vi "RT Driver VI.vi"(7 "Operation":T1, 11 "Device Reference in":T2 format="%.0x") -> (0 "Error Code":i32)   [LabVIEW 2013, in "FPGA Addon Engine.lvlib"]
uses:
  FPGA Addon Engine.lvlib
  <vilib>/NI Veristand/Custom Device API/Custom Device Item Ref.ctl
  <vilib>/NI Veristand/Custom Device API/Hardware Interface Driver VI Operation.ctl
  Shared/FPGA Settings.vi
  SubVIs/Initialize Scalar Datatypes and Refs.vi
  <vilib>/Utility/config.llb/Open Config Data.vi
  <vilib>/Utility/config.llb/Get Key Names.vi
  <vilib>/Utility/config.llb/Write Key.vi
  <vilib>/Utility/config.llb/Write Key (I32).vi
  <vilib>/Utility/config.llb/Close Config Data.vi
  Shared/Constants.vi
  <vilib>/NI Veristand/Custom Device API/NI VeriStand - Get Item Property.vi
  <vilib>/NI Veristand/Custom Device API/Get Item Property (Variant).vi
  <vilib>/NI Veristand/Custom Device API/NI VeriStand - Get Target Type.vi
  <vilib>/NI Veristand/Custom Device API/Get Item Property (Dependent File).vi
  SubVIs/Initialize Input DMA Refs.vi
  SubVIs/Initialize Output DMA Refs.vi
  <vilib>/NI Veristand/Custom Device API/Get Item Property (Path).vi
  <vilib>/NI Veristand/Custom Device API/Get Item Property (String).vi
  SubVIs/Initialize Scalar Datatype Classes.vi
  SubVIs/Output DMA Engine.vi
  <vilib>/rvi/interface/common/niFpgaWaitOnOcc.vi
  <vilib>/Utility/error.llb/Error Cluster From Error Code.vi
  <vilib>/RVI Host/nirviSupport.llb/nirviErrorClusterFromErrorCode.vi
  <vilib>/rvi/errors/niLvFpgaAdjustHostInterfaceError.vi
  <vilib>/NI Veristand/Custom Device API/Global Data Refs.vi
  <vilib>/FPGAPlugInAG/Dynamic/niLvFpga_Close_Dynamic.vi
  <vilib>/NI Veristand/Custom Device Waveform API/Multiple Waveforms Write (DBL)/Multiple Waveforms Write (DBL).lvclass
  <vilib>/NI Veristand/Custom Device Waveform API/Single Waveform Read (DBL)/Single Waveform Read (DBL).lvclass
  <vilib>/rvi/interface/nirviMethod/nirviMethod.xnode
  <vilib>/rvi/interface/nirviCloseFPGA/nirviCloseFPGA.xnode
  <vilib>/NI VeriStand/Custom Device API/Custom Device API.lvlib
  <vilib>/NI Veristand/Custom Device Tools/Custom Device Utility Library/Custom Device Utility Library.lvlib
  SubVIs/Inline Async API/Inline Async API.lvlib
  SubVIs/Error Handling API/Error Handling API.lvlib
  <vilib>/rvi/interface/nirviMethod/StockFPGA_InlinedMethodWaitForSingleIRQ.vi
  <vilib>/FPGAPlugInAG/Dynamic/niLvFpga_WaitOnIrq_Dynamic.vi
  <vilib>/FPGAPlugInAG/Dynamic/niLvFpga_AcknowledgeIrq_Dynamic.vi
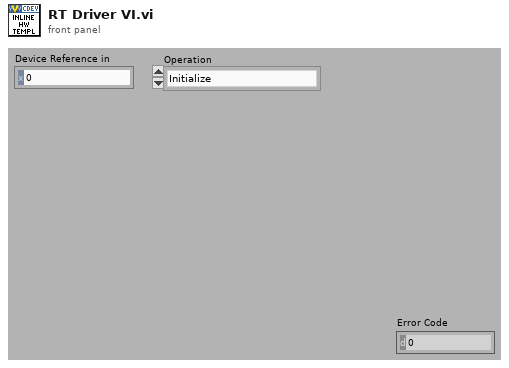
[diagram p1: front panel]
types:
  T1 = typedef "Custom Device API.lvlib/Hardware Interface Driver VI Operation.ctl" = enum16{"Initialize", "Start", "Read Data from HW", "Write Data to HW", "Close"}
  T2 = typedef "Custom Device API.lvlib/Custom Device Item Ref.ctl" = u64
  T3 = typedef "FPGA Addon Engine.lvlib/State Variables.ctl" = cluster{"FPGA Ref":refnum<k20>, "IncomingRegisters.Refs":T4[], "IncomingDMA.Refs":T7[], "OutgoingRegisters.Refs":T4[], "OutgoingDMA.Refs":T12[], "Compiled":T14}
  T4 = typedef "FPGA Addon Engine.lvlib/Register Settings.ctl" = cluster{"Data Type":T5, "U64":refnum<k20>, "U32":refnum<k20>, "U16":refnum<k20>, "U8":refnum<k20>, "I64":refnum<k20>, "I32":refnum<k20>, "I16":refnum<k20>, "I8":refnum<k20>, "SGL":refnum<k20>, "Bool":refnum<k20>, "Scalar Type":T6, "Index":i32, "Length":i32}
  T5 = typedef "Type Descriptor Enumeration__ogtk.ctl" = enum8{"<Null>", "I8", "I16", "I32", "I64", "U8", "U16", "U32", "U64", "SGL", "DBL", "EXT", "CSG", "CDB", "CXT", "0x0F", "0x10", "0x11", "0x12", "0x13", "0x14", "Enum U8", "Enum U16", "Enum U32", "Enum U64", "SGL PQ", "DBL PQ", "EXT PQ", "CSG PQ", "CDB PQ", "CXT PQ", "0x1F", "0x20", "Boolean", "0x22", "0x23", "0x24", "0x25", "0x26", "0x27", "0x28", "0x29", "0x2A", "0x2B", "0x2C", "0x2D", "0x2E", "0x2F", "String", "0x31", "Path", "Pict", "0x34", "0x35", "0x36", "DAQ", "0x38", "0x39", "0x3A", "0x3B", "0x3C", "0x3D", "0x3E", "0x3F", "Array", "0x41", "0x42", "0x43", "0x44", "0x45", "0x46", "0x47", "0x48", "0x49", "0x4A", "0x4B", "0x4C", "0x4D", "0x4E", "0x4F", "Cluster", "0x51", "0x52", "Variant", "Waveform", "0x55", "0x56", "0x57", "0x58", "0x59", "0x5A", "0x5B", "0x5C", "0x5D", "0x5E", "0x5F", "0x60", "0x61", "0x62", "0x63", "0x64", "0x65", "0x66", "0x67", "0x68", "0x69", "0x6A", "0x6B", "0x6C", "0x6D", "0x6E", "0x6F", "Refnum"}
  T6 = typedef "FPGA Addon Shared.lvlib/Scalar Type.ctl" = enum16{"Standard", "Bitpacked"}
  T7 = typedef "FPGA Addon Engine.lvlib/DMA Input References.ctl" = cluster{"Waveform Ref":refnum<class "Multiple Waveforms Write (DBL).lvclass">, "DMA Ref":T8, "Write to VS Engine.Refs":cluster{"Refs":T9[], "Values":dbl[]}, "Write to VS Engine.FIFO":refnum<k33>, "Name":string, "DMA Settings":T10}
  T8 = typedef "FPGA Addon Engine.lvlib/DMA Input Ref.ctl" = refnum<k20>
  T9 = typedef "Custom Device API.lvlib/Data Reference.ctl" = i32
  T10 = typedef "FPGA Addon Shared.lvlib/DMA Settings.ctl" = cluster{"Number of Channels":u8, "Delacing Scheme":T11, "Update Rate":u32, "dt":dbl}
  T11 = typedef "FPGA Addon Shared.lvlib/Delacing Scheme.ctl" = enum8{"Interlaced"}
  T12 = typedef "FPGA Addon Engine.lvlib/DMA Output References.ctl" = cluster{"Write to VS Engine.Refs":cluster{"Refs":T9[], "Values":dbl[]}, "Waveforms":refnum<class "Single Waveform Read (DBL).lvclass">[], "DMA Ref":T13, "Write to VS Engine.FIFO":refnum<k33>, "Name":string}
  T13 = typedef "FPGA Addon Engine.lvlib/DMA Output Ref.ctl" = refnum<k20>
  T14 = typedef "FPGA Addon Shared.lvlib/Compiled.Settings" = cluster{"Name":string, "IncomingRegisters.Settings":T15[], "IncomingRegisters.Refs":cluster{"Refs":T17[], "Values":dbl[]}, "OutgoingRegisters.Settings":T15[], "OutgoingRegisters.Refs":cluster{"Refs":T17[], "Values":dbl[]}, "Incoming.Size":i32, "Outgoing.Size":i32, "IncomingDMA.Settings":T18[], "OutgoingDMA.Settings":T18[], "FPGA.Settings":T20}
  T15 = typedef "FPGA Addon Shared.lvlib/Compiled.RegisterSettings.ctl" = cluster{"Scalar Type":T6, "Index":i32, "Length":i32, "Register":T16}
  T16 = typedef "FPGA Addon Shared.lvlib/Register Information.ctl" = cluster{"Name":string, "Data Type":T5, "Default Value":dbl}
  T17 = typedef "Custom Device API.lvlib/Block Data Reference.ctl" = cluster{"Data Reference":T9, "Offset":i32, "Length":i32}
  T18 = typedef "FPGA Addon Shared.lvlib/Compiled.DMASettings.ctl" = cluster{"Name":string, "DMA.Settings":T10, "DMA.VSRefs":T19[], "WritetoVSEngine.Refs":cluster{"Refs":T9[], "Values":dbl[]}}
  T19 = typedef "Custom Device API.lvlib/Waveform Data Reference.ctl" = i32
  T20 = typedef "FPGA Addon Shared.lvlib/FPGA Settings.ctl" = cluster{"Bitfile path":path, "RIO Device Address":string}
  T21 = typedef "FPGA Addon Engine.lvlib/Error Handling API.lvlib/Error Handling Cluster.ctl" = cluster{"Error Process Q":refnum<queue>, "Process Qs":refnum<queue>[]}
  T22 = cluster{"Vars":T3, "Async?":bool, "Async VI Refs out":refnum<vi>[], "Error Handling Refs":T21, "error out":errorcluster}
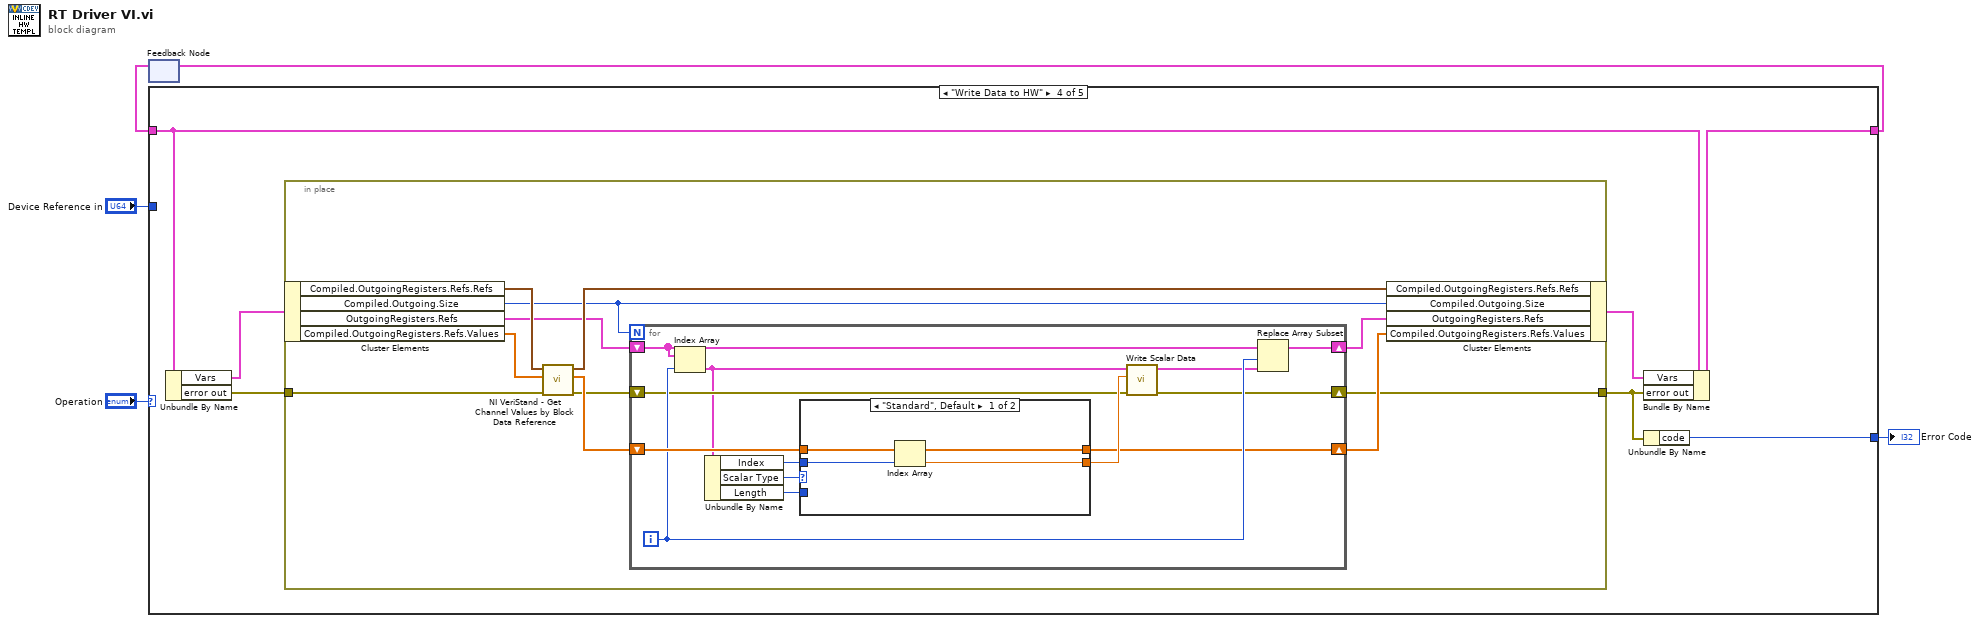
[diagram p0: block diagram]
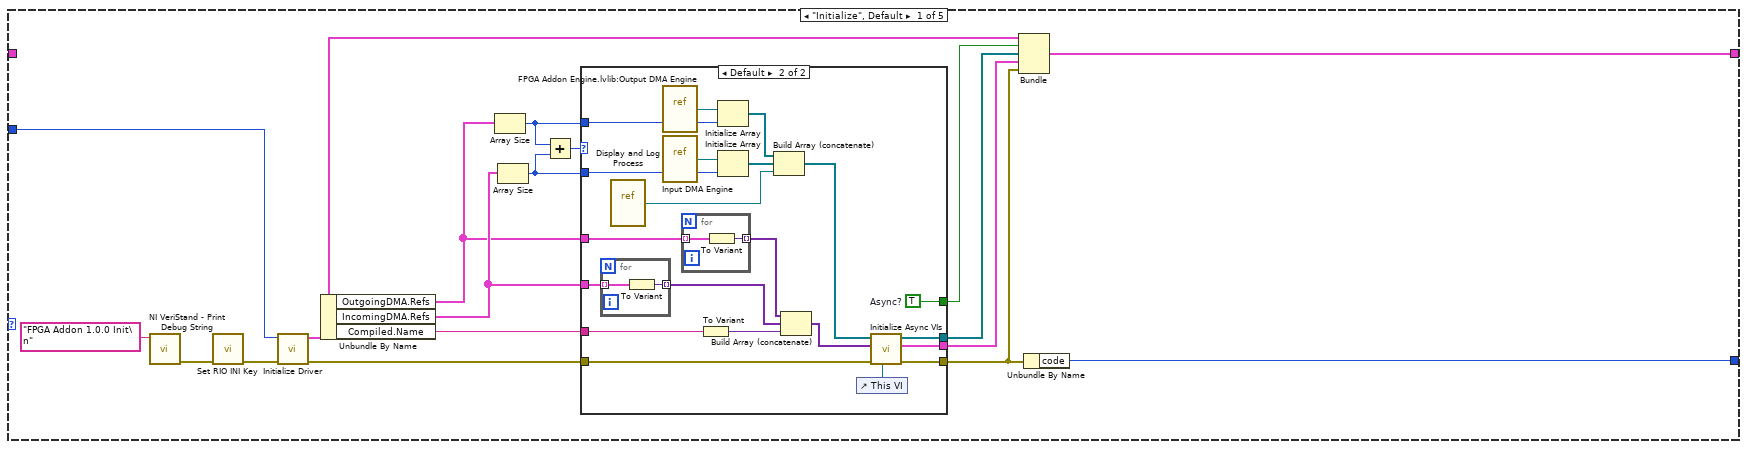
[diagram p2: hidden frame]
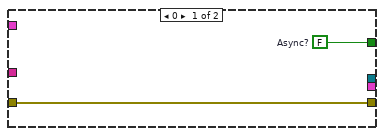
[diagram p3: hidden frame]
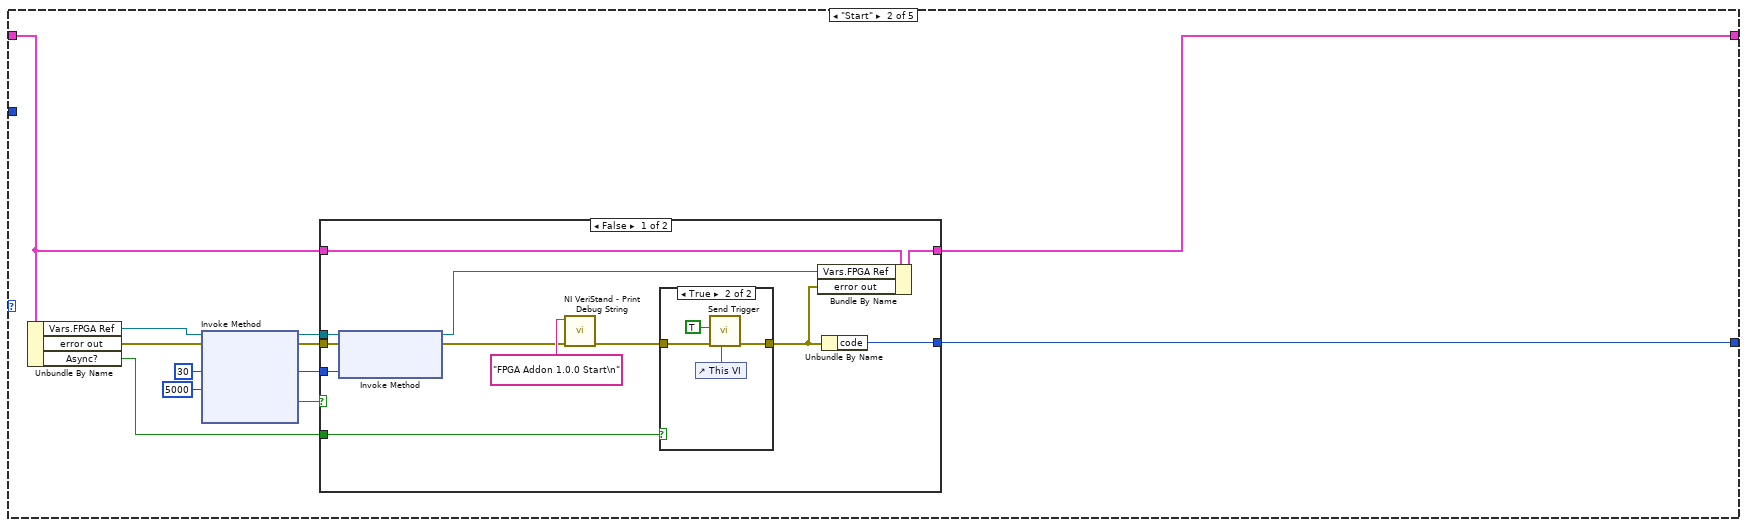
[diagram p4: hidden frame]
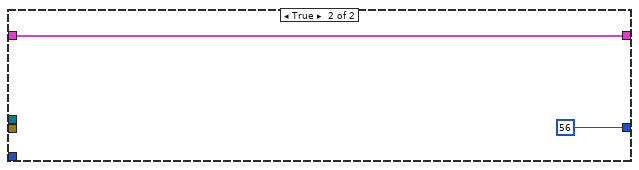
[diagram p6: hidden frame]
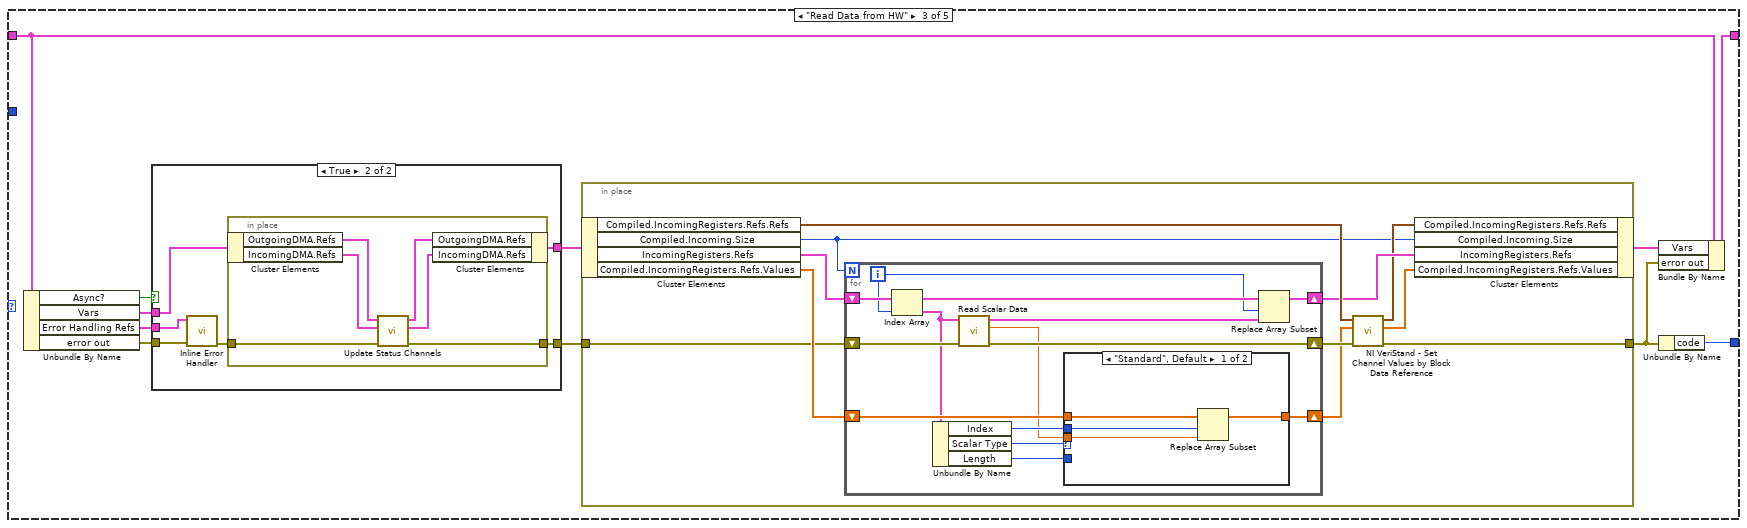
[diagram p7: hidden frame]
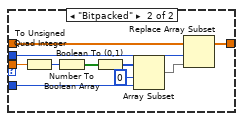
[diagram p9: hidden frame]
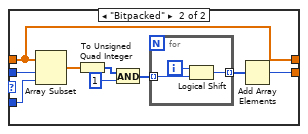
[diagram p10: hidden frame]
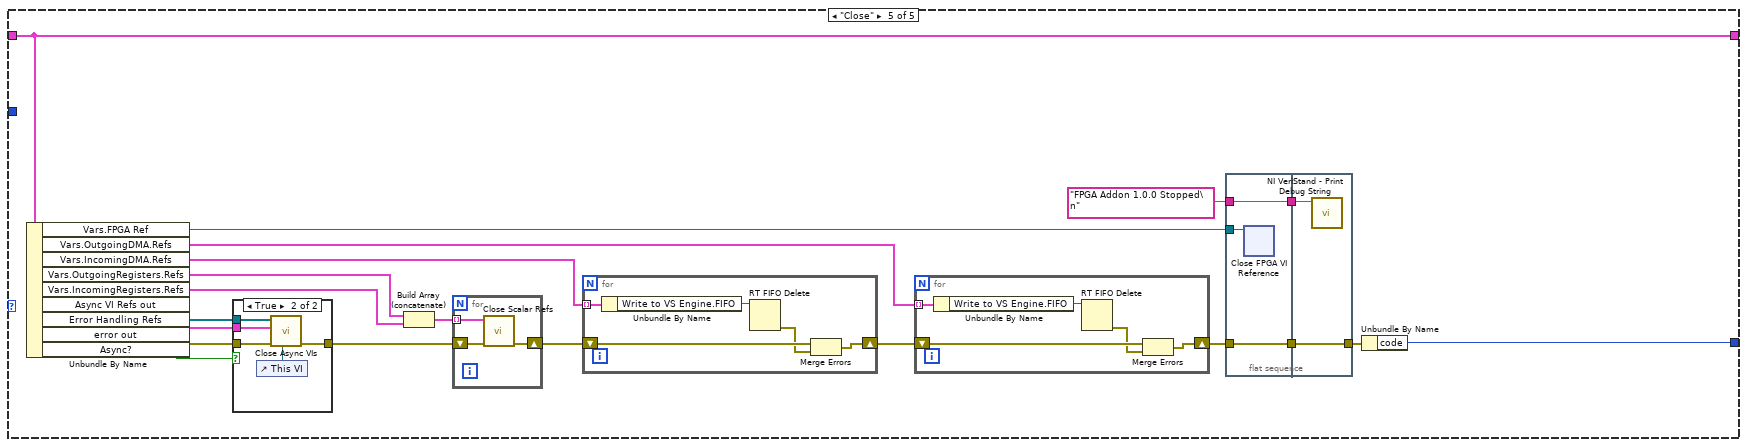
[diagram p11: hidden frame]
diagram:
  n1 = feedback #1() -> (w3:T22)  [unwired: 1 out]
  n2 = case shown="\"Write Data to HW\"" "Operation" {
    tunnel: [w23 w59 w89 w144 w207] -> w4
    tunnel: w3 -> [_ w60 w90 w145 w207]
    tunnel: "Device Reference in" -> [w21 _ _ _ _]
    tunnel: [w22 w61 w87 w146 w209] -> w1
    frame "Initialize", Default {
      n3 = call <vilib>:"NI VeriStand - Print Debug String.vi"("Message"="FPGA Addon 1.0.0 Init\n") -> ("error out"=w19:errorcluster)  [unwired: 10 in]
      n4 = call "Set RIO INI Key.vi"("error in (no error)"=w19) -> ("error out"=w18:errorcluster)  [unwired: 10 in]
      n5 = call "Initialize Driver.vi"("error in (no error)"=w18, "Section Ref in"=w21) -> ("error out"=w17:errorcluster, "Vars"=w6:T3)  [unwired: 8 in]
      n6 = Unbundle By Name(w6) -> ("OutgoingDMA.Refs"=w11:T12[], "IncomingDMA.Refs"=w13:T7[], "Compiled.Name"=w12:string)
      n7 = Array Size(array=w11) -> (size(s)=w10:i32)
      n8 = Array Size(array=w13) -> (size(s)=w9:i32)
      n9 = Add(x=w10, y=w9) -> (x+y=w8:i32)
      n10 = case shown="Default" w8 {
        tunnel: w17 -> [w25 w46]
        tunnel: [w25 w45] -> w16
        tunnel: [_ w40] -> w15
        tunnel: [_ w39] -> w14
        tunnel: w13 -> [_ w37]
        tunnel: w12 -> [_ w33]
        tunnel: w11 -> [_ w30]
        tunnel: w10 -> [_ w28]
        tunnel: w9 -> [_ w27]
        tunnel: [w24 w26] -> w7
        frame 0 {
          w24 = FALSE  # Async?
        }
        frame Default {
          w26 = TRUE  # Async?
          n11 = for {
            tunnel: w37 -> [w50] mode=indexing
            tunnel: [w49] -> w36 mode=indexing
            n12 = To Variant(anything=w50) -> (Variant=w49:variant)
          }
          n13 = vi-ref "Display and Log Process.vi"() -> (w41:refnum<vi>)
          n14 = vi-ref "FPGA Addon Engine.lvlib:Output DMA Engine.vi"() -> (w32:refnum<vi>)
          n15 = vi-ref "Input DMA Engine.vi"() -> (w44:refnum<vi>)
          n16 = for {
            tunnel: w30 -> [w48] mode=indexing
            tunnel: [w47] -> w29 mode=indexing
            n17 = To Variant(anything=w48) -> (Variant=w47:variant)
          }
          n18 = To Variant(anything=w33) -> (Variant=w35:variant)
          n19 = Initialize Array(w32, w28) -> (w31:refnum<vi>[])
          n20 = Initialize Array(w44, w27) -> (w43:refnum<vi>[])
          n21 = Build Array (concatenate)(w31, w43, w41) -> (w42:refnum<vi>[])
          n22 = Build Array (concatenate)(w29, w36, w35) -> (w34:variant[])
          n23 = control-ref of="This VI"() -> (w38:refnum<vi>)
          n24 = call "Initialize Async VIs.vi"("VI in"=w38, "error in (no error)"=w46, "Async VI Parameters"=w34, "Async VI Refs"=w42) -> ("error out"=w45:errorcluster, "Error Handling Refs"=w40:T21, "Async VI Refs out"=w39:refnum<vi>[])  [unwired: 5 in]
        }
      }
      n25 = Bundle("Vars"=w6, "Async?"=w7, "Async VI Refs out"=w14, "Error Handling Refs"=w15, "error out"=w16) -> (w23:T22)  [unwired: 1 out]
      n26 = Unbundle By Name(w16) -> ("code"=w22:i32)
    }
    frame "Start" {
      w54 = 30 ("IRQ Number(s)")
      n27 = Unbundle By Name(w60) -> ("Vars.FPGA Ref"=w58:refnum<k20>, "error out"=w57:errorcluster, "Async?"=w52:bool)
      n28 = xnode "Invoke Method"("FPGA VI Reference In"=w58, "error in"=w57, "IRQ Number(s)"=w54, "Timeout (ms)"=5000) -> ("FPGA VI Reference Out"=w56:refnum<k20>, "error out"=w55:errorcluster, "Timed Out"=w51:bool)  [unwired: 1 out]
      n29 = case shown="False" w51 {
        tunnel: [w73 56 ("code")] -> w61
        tunnel: w60 -> [w72 w80]
        tunnel: [w71 w80] -> w59
        tunnel: w56 -> [w69 _]
        tunnel: w55 -> [w68 _]
        tunnel: w54 -> [w67 _]
        tunnel: w52 -> [w62 _]
        frame False {
          n30 = xnode "Invoke Method"("FPGA VI Reference In"=w69, "error in"=w68, "IRQ Number(s)"=w67) -> ("FPGA VI Reference Out"=w66:refnum<k20>, "error out"=w65:errorcluster)
          n31 = call <vilib>:"NI VeriStand - Print Debug String.vi"("error in (no error)"=w65, "Message"="FPGA Addon 1.0.0 Start\n") -> ("error out"=w64:errorcluster)  [unwired: 9 in]
          n32 = case shown="True" w62 {
            tunnel: w64 -> [w74 w76]
            tunnel: [w74 w75] -> w63
            frame False {
            }
            frame True {
              n33 = control-ref of="This VI"() -> (w78:refnum<vi>)
              n34 = call "Send Trigger.vi"("Parent VI"=w78, "error in (no error)"=w76, "notification"=TRUE) -> ("error out"=w75:errorcluster)  [unwired: 8 in]
            }
          }
          n35 = Bundle By Name(cluster=w72, "Vars.FPGA Ref"=w66, "error out"=w63) -> (w71:T22)
          n36 = Unbundle By Name(w63) -> ("code"=w73:i32)
        }
        frame True {
        }
      }
    }
    frame "Read Data from HW" {
      n37 = Unbundle By Name(w90) -> ("Async?"=w81:bool, "Vars"=w84:T3, "Error Handling Refs"=w85:T21, "error out"=w86:errorcluster)
      n38 = case shown="True" w81 {
        tunnel: w86 -> [w93 w99]
        tunnel: w85 -> [_ w98]
        tunnel: w84 -> [w92 w97]
        tunnel: [w92 w96] -> w83
        tunnel: [w93 w94] -> w82
        frame False {
        }
        frame True {
          n39 = call "Inline Error Handler.vi"("error in"=w99, "Error Handling Cluster"=w98) -> ("error out"=w95:errorcluster)  [unwired: 9 in]
          n40 = in-place {
            in-place-border: [w101] -> w94
            in-place-border: w95 -> [w100]
            n41 = in-place-cluster #2(w97) -> ("OutgoingDMA.Refs"=w103:T12[], "IncomingDMA.Refs"=w105:T7[])
            n42 = call "Update Status Channels.vi"("error in (no error)"=w100, "DMA Input Settings"=w105, "DMA Output Settings"=w103) -> ("error out"=w101:errorcluster, "DMA Input Settings"=w104:T7[], "DMA Output Settings"=w102:T12[])  [unwired: 6 in]
            n43 = in-place-cluster #2("OutgoingDMA.Refs"=w102, "IncomingDMA.Refs"=w104) -> (w96:T3)
          }
        }
      }
      n44 = in-place {
        in-place-border: w82 -> [w107]
        in-place-border: [w109] -> w88
        n45 = in-place-cluster #3(w83) -> ("Compiled.IncomingRegisters.Refs.Refs"=w113:T17[], "Compiled.Incoming.Size"=w108:i32, "IncomingRegisters.Refs"=w116:T4[], "Compiled.IncomingRegisters.Refs.Values"=w115:dbl[])
        n46 = for {
          N: w108 -> [_]
          shift-right: [w128] -> w106
          shift-left: w115 -> [w129]
          shift-right: [w127] -> w112
          shift-left: w116 -> [w126]
          shift-right: [w124] -> w114
          shift-left: w107 -> [w125]
          i -> [w119]
          n47 = Index Array(array=w126, index=w119) -> (element=w122:T4)
          n48 = Unbundle By Name(w122) -> ("Index"=w120:i32, "Scalar Type"=w121:T6, "Length"=w118:i32)
          n49 = call "Read Scalar Data.vi"("error in (no error)"=w125, "Cluster"=w122) -> ("error out"=w124:errorcluster, "Value"=w117:dbl, "Cluster"=w123:T4)  [unwired: 7 in]
          n50 = case shown="\"Standard\", Default" w121 {
            tunnel: w129 -> [w133 w138]
            tunnel: [w132 w137] -> w128
            tunnel: w117 -> [w131 w143]
            tunnel: w120 -> [w130 w135]
            tunnel: w118 -> [_ w139]
            frame "Standard", Default {
              n51 = Replace Array Subset(array=w133, new element=w131, index=w130) -> (w132:dbl[])
            }
            frame "Bitpacked" {
              n52 = To Unsigned Quad Integer(1:w143) -> (0:w141:u64)
              n53 = Number To Boolean Array(number=w141) -> (Boolean array=w142:bool[])
              n54 = Boolean To (0,1)(Boolean=w142) -> (0, 1=w140:i16[])
              n55 = Array Subset(array=w140, index=0, length=w139) -> (w136:i16[])
              n56 = Replace Array Subset(array=w138, new element=w136, index=w135) -> (w137:dbl[])
            }
          }
          n57 = Replace Array Subset(array=w126, new element=w123, index=w119) -> (w127:T4[])
        }
        n58 = call <vilib>:"NI VeriStand - Set Channel Values by Block Data Reference.vi"("error in (no error)"=w114, "Values Array in"=w106, "Block Data Ref"=w113) -> ("error out"=w109:errorcluster, "Values Array out"=w110:dbl[], "Block Data Ref dup"=w111:T17[])  [unwired: 6 in]
        n59 = in-place-cluster #3("Compiled.IncomingRegisters.Refs.Refs"=w111, "Compiled.Incoming.Size"=w108, "IncomingRegisters.Refs"=w112, "Compiled.IncomingRegisters.Refs.Values"=w110) -> (w91:T3)
      }
      n60 = Bundle By Name(cluster=w90, "Vars"=w91, "error out"=w88) -> (w89:T22)
      n61 = Unbundle By Name(w88) -> ("code"=w87:i32)
    }
    frame "Write Data to HW" {
      n62 = Unbundle By Name(w145) -> ("Vars"=w149:T3, "error out"=w147:errorcluster)
      n63 = in-place {
        in-place-border: w147 -> [w152]
        in-place-border: [w155] -> w150
        n64 = in-place-cluster #4(w149) -> ("Compiled.OutgoingRegisters.Refs.Refs"=w161:T17[], "Compiled.Outgoing.Size"=w157:i32, "OutgoingRegisters.Refs"=w159:T4[], "Compiled.OutgoingRegisters.Refs.Values"=w154:dbl[])
        n65 = call <vilib>:"NI VeriStand - Get Channel Values by Block Data Reference.vi"("error in (no error)"=w152, "Values Array in"=w154, "Block Data Ref"=w161) -> ("error out"=w151:errorcluster, "Values Array out"=w153:dbl[], "Block Data Ref dup"=w160:T17[])  [unwired: 6 in]
        n66 = for {
          N: w157 -> [_]
          shift-right: [w162] -> w156
          shift-left: w153 -> [w172]
          shift-right: [w174] -> w158
          shift-left: w159 -> [w173]
          shift-right: [w167] -> w155
          shift-left: w151 -> [w168]
          i -> [w171]
          n67 = Index Array(array=w173, index=w171) -> (element=w166:T4)
          n68 = Unbundle By Name(w166) -> ("Index"=w164:i32, "Scalar Type"=w165:T6, "Length"=w163:i32)
          n69 = case shown="\"Standard\", Default" w165 {
            tunnel: w172 -> [w175 w178]
            tunnel: w164 -> [w177 w186]
            tunnel: [w176 w179] -> w170
            tunnel: w163 -> [_ w185]
            tunnel: [w175 w178] -> w162
            frame "Standard", Default {
              n70 = Index Array(array=w175, index=w177) -> (element=w176:dbl)
            }
            frame "Bitpacked" {
              n71 = Array Subset(array=w178, index=w186, length=w185) -> (w180:dbl[])
              n72 = To Unsigned Quad Integer(1:w180) -> (0:w181:u64[])
              n73 = And(x=w181, y=u64 1) -> (x .and. y?=w183:u64[])
              n74 = for {
                tunnel: w183 -> [w189] mode=indexing
                tunnel: [w187] -> w184 mode=indexing
                i -> [w188]
                n75 = Logical Shift(y=w188, x=w189) -> (x << y=w187:u64)
              }
              n76 = Add Array Elements(numeric array=w184) -> (sum=w179:u64)
            }
          }
          n77 = call "Write Scalar Data.vi"("error in (no error)"=w168, "Value"=w170, "Cluster"=w166) -> ("error out"=w167:errorcluster, "Cluster"=w169:T4)  [unwired: 7 in]
          n78 = Replace Array Subset(array=w173, new element=w169, index=w171) -> (w174:T4[])
        }
        n79 = in-place-cluster #4("Compiled.OutgoingRegisters.Refs.Refs"=w160, "Compiled.Outgoing.Size"=w157, "OutgoingRegisters.Refs"=w158, "Compiled.OutgoingRegisters.Refs.Values"=w156) -> (w148:T3)
      }
      n80 = Bundle By Name(cluster=w145, "Vars"=w148, "error out"=w150) -> (w144:T22)
      n81 = Unbundle By Name(w150) -> ("code"=w146:i32)
    }
    frame "Close" {
      n82 = Unbundle By Name(w207) -> ("Vars.FPGA Ref"=w196:refnum<k20>, "Vars.OutgoingDMA.Refs"=w190:T12[], "Vars.IncomingDMA.Refs"=w195:T7[], "Vars.OutgoingRegisters.Refs"=w206:T4[], "Vars.IncomingRegisters.Refs"=w205:T4[], "Async VI Refs out"=w202:refnum<vi>[], "Error Handling Refs"=w201:T21, "error out"=w204:errorcluster, "Async?"=w193:bool)
      n83 = case shown="True" w193 {
        tunnel: w204 -> [w215 w220]
        tunnel: [w215 w219] -> w203
        tunnel: w202 -> [_ w218]
        tunnel: w201 -> [_ w217]
        frame False {
        }
        frame True {
          n84 = control-ref of="This VI"() -> (w216:refnum<vi>)
          n85 = call "Close Async VIs.vi"("TopLevel VI"=w216, "error in (no error)"=w220, "Error Handling Refs"=w217, "Async VI"=w218) -> ("error out"=w219:errorcluster)  [unwired: 7 in]
        }
      }
      n86 = Build Array (concatenate)(w206, w205) -> (w208:T4[])
      n87 = for {
        tunnel: w208 -> [w231] mode=indexing
        shift-right: [w232] -> w194
        shift-left: w203 -> [w233]
        n88 = call "Close Scalar Refs.vi"("error in (no error)"=w233, "Cluster"=w231) -> ("error out"=w232:errorcluster)  [unwired: 9 in]
      }
      n89 = for {
        shift-right: [w221] -> w192
        shift-left: w194 -> [w223]
        tunnel: w195 -> [w225] mode=indexing
        n90 = Unbundle By Name(w225) -> ("Write to VS Engine.FIFO"=w224:refnum<k33>)
        n91 = RT FIFO Delete(0:w224) -> (11:w222:errorcluster)  [unwired: 2 in]
        n92 = Merge Errors(w223, w222) -> (w221:errorcluster)
      }
      n93 = for {
        shift-right: [w210] -> w191
        shift-left: w192 -> [w212]
        tunnel: w190 -> [w214] mode=indexing
        n94 = Unbundle By Name(w214) -> ("Write to VS Engine.FIFO"=w213:refnum<k33>)
        n95 = RT FIFO Delete(0:w213) -> (11:w211:errorcluster)  [unwired: 2 in]
        n96 = Merge Errors(w212, w211) -> (w210:errorcluster)
      }
      n97 = flat-sequence {
        tunnel: "FPGA Addon 1.0.0 Stopped\n" -> [w227]
        tunnel: w191 -> [w228]
        tunnel: [w228] -> w198
        tunnel: [w227] -> w197
        tunnel: w196 -> [w226]
        tunnel: [w230] -> w200
        tunnel: w198 -> [w230]
        tunnel: w197 -> [w229]
        frame #0 {
          n98 = xnode "Close FPGA VI Reference"("FPGA VI Reference In"=w226) -> ()  [unwired: 1 in, 1 out]
        }
        frame #1 {
          n99 = call <vilib>:"NI VeriStand - Print Debug String.vi"("Message"=w229) -> ()  [unwired: 10 in, 1 out]
        }
      }
      n100 = Unbundle By Name(w200) -> ("code"=w209:i32)
    }
  }
  "Error Code" <- w1
  n101 = feedback-in #1(w4) -> ()
